vi "sem.Release.vi"(8 "error in":errorcluster, 11 "camera.nit in":refnum<class "camera.lvclass">) -> (0 "error out":errorcluster)   [LabVIEW 2020, in "camera.lvclass"]
uses:
  camera.lvclass
  camera.lvclass/camera.ctl
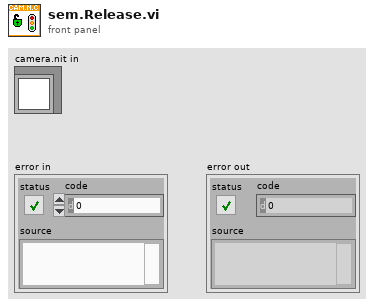
[diagram p1: front panel]
types:
  T1 = typedef "Semaphore RefNum" = refnum<k1>
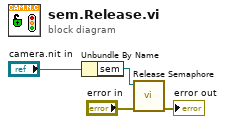
[diagram p0: block diagram]
diagram:
  n1 = Unbundle By Name("camera.nit in") -> ("sem"=w2:T1)
  n2 = call <vilib>:"Release Semaphore.vi"("error in (no error)"="error in", "semaphore"=w2) -> ("error out"=→"error out":errorcluster)  [unwired: 4 in, 1 out]
